vi "STM Get Connection Reference (TCP).vi"(8 "error in":errorcluster, 11 "Connection Info":T1) -> (0 "error out":errorcluster, 2 "connection ID out":refnum<k5>, 3 "Connection Info Out":T1)   [LabVIEW 2010]
doc: "Returns the TCP/IP connection reference."
uses:
  stm_TCP Connection Info.ctl
  stm_MetaDataElement.ctl
  NI STM.lvlib
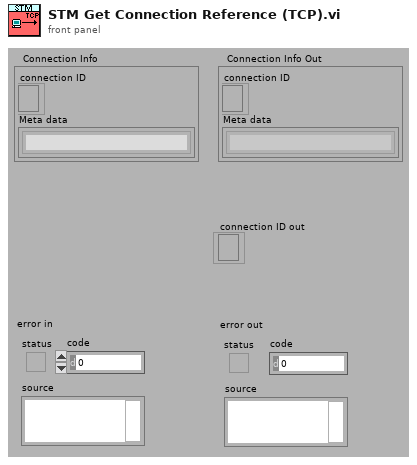
[diagram p1: front panel]
types:
  T1 = typedef "stm_TCP Connection Info.ctl" = cluster{"connection ID":refnum<k5>, "Meta data":T2[]}
  T2 = typedef "stm_MetaDataElement.ctl" = string
  T3 = typedef "NI STM.lvlib/TCP Connection Info.ctl" = cluster{"connection ID":refnum<k5>, "Meta data":T4[]}
  T4 = typedef "NI STM.lvlib/MetaDataElement.ctl" = string
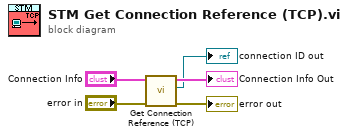
[diagram p0: block diagram]
diagram:
  n1 = call "Get Connection Reference (TCP).vi"("error in"="error in", "Connection Info"="Connection Info") -> ("error out"=→"error out":errorcluster, "connection ID out"=→"connection ID out":refnum<k5>, "Connection Info Out"=→"Connection Info Out":T3)  [unwired: 7 in]
